vi "niFpgaMemoryEmulationDramRetrieveData.vi"(0 "fifo size":u32, 1 "name":string, 5 "ref in wired":bool, 7 "data type":i32, 9 "ready for output":bool, 11 "error in (no error)":errorcluster) -> (8 "data":i32, 10 "output valid":bool, 15 "error out":errorcluster)   [LabVIEW 2017]
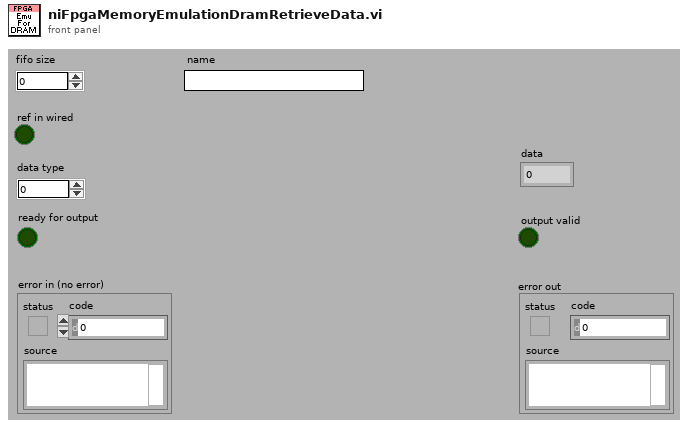
[diagram p1: front panel]
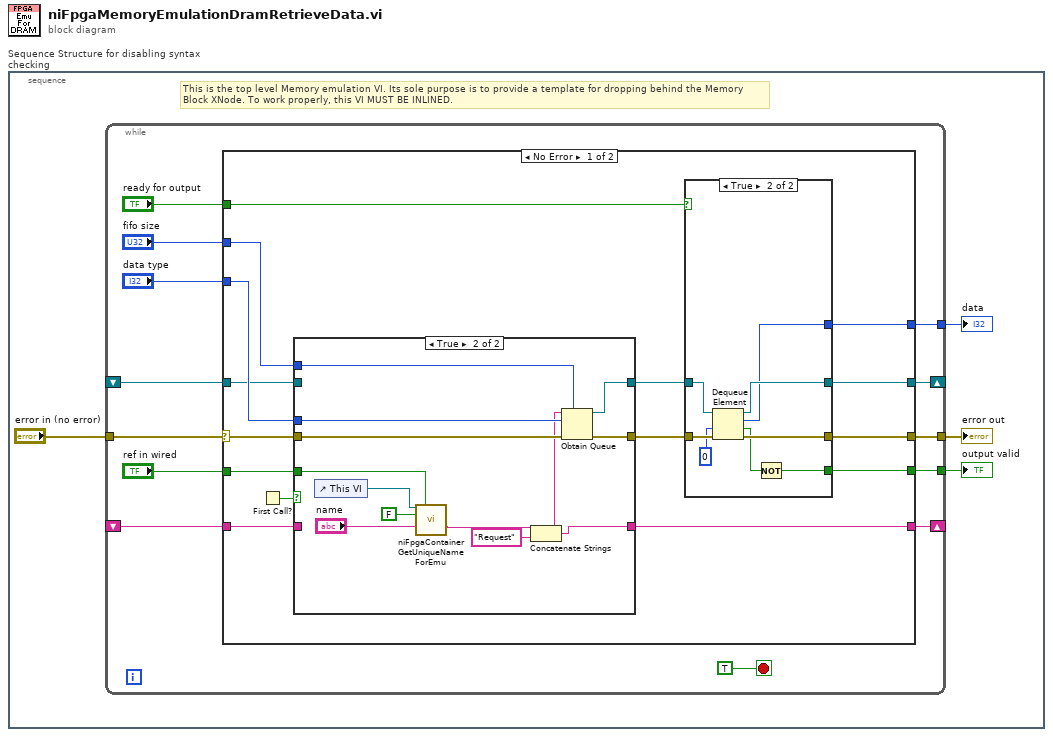
[diagram p0: block diagram]
diagram:
  n1 = stacked-sequence "Sequence Structure for disabling syntax checking" {
    frame #0 {
      # "This is the top level Memory emulation VI. Its sole purpose is to provide a template for dropping behind the Memory Block XNode. To work properly, this VI MUST BE INLINED."
      n2 = while {
        shift-right: [w15] -> _
        shift-left: _ -> [w17]
        tunnel: [w14] -> w1
        tunnel: "error in (no error)" -> [w13]
        tunnel: [w10] -> w3
        shift-right: [w8] -> _
        shift-left: _ -> [w7]
        tunnel: [w6] -> w4
        stop <- TRUE stop-if-true
        n3 = case shown="No Error" w13 {
          selector: w13 -> [w29 w60]
          tunnel: w17 -> [w25 w59]
          tunnel: [w31 w59] -> w15
          tunnel: [w21 w60] -> w14
          tunnel: "ref in wired" -> [w32 _]
          tunnel: "ready for output" -> [w24 _]
          tunnel: [w18 _] -> w10
          tunnel: "fifo size" -> [w28 _]
          tunnel: [w20 w58] -> w8
          tunnel: w7 -> [w26 w58]
          tunnel: [w19 _] -> w6
          tunnel: "data type" -> [w27 _]
          frame No Error {
            n4 = First Call?() -> (First Call?: T/F=w30:bool)
            n5 = case shown="True" w30 {
              tunnel: w32 -> [_ w57]
              tunnel: [w44 w46] -> w31
              tunnel: w29 -> [w43 w53]
              tunnel: w28 -> [_ w52]
              tunnel: w27 -> [_ w51]
              tunnel: [w45 w50] -> w22
              tunnel: w26 -> [w45 _]
              tunnel: [w43 w49] -> w23
              tunnel: w25 -> [w44 _]
              frame False {
              }
              frame True {
                n6 = control-ref of="This VI"() -> (w55:refnum<vi>)
                n7 = call <vilib>:"niFpgaContainerGetUniqueNameForEmu.vi"("parent VI"=w55, "ref in wired"=w57, "local"=FALSE, "name in"="name") -> ("name out"=w47:string)  [unwired: 11 in]
                n8 = Concatenate Strings(w47, "Request" ("string")) -> (w46:string)
                n9 = Obtain Queue(max queue size (-1, unlimited)=w52, name (unnamed)=w46, element data type=w51, error in (no error)=w53) -> (queue out=w50:refnum<queue>, error out=w49:errorcluster)  [unwired: 1 in, 1 out]
              }
            }
            n10 = case shown="True" w24 {
              tunnel: w23 -> [w34 w42]
              tunnel: w22 -> [w33 w41]
              tunnel: [w34 w39] -> w21
              tunnel: [w33 w38] -> w20
              tunnel: [_ w37] -> w19
              tunnel: [_ w35] -> w18
              frame False {
              }
              frame True {
                n11 = Dequeue Element(queue=w41, timeout in ms (-1)=0, error in (no error)=w42) -> (queue out=w38:refnum<queue>, element=w37:i32, timed out?=w36:bool, error out=w39:errorcluster)
                n12 = Not(x=w36) -> (.not. x?=w35:bool)
              }
            }
          }
          frame Error {
          }
        }
      }
      "error out" <- w1
      "output valid" <- w3
      "data" <- w4
    }
  }
